vi "IDCheck.vi"(10 "IDIn":u8) -> (2 "IDOut":u8)   [LabVIEW 2013]
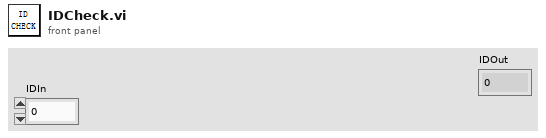
[diagram p1: front panel]
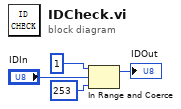
[diagram p0: block diagram]
diagram:
  n1 = In Range and Coerce(upper limit=u8 1, x="IDIn", lower limit=u8 253) -> (coerced(x)=→"IDOut":u8)  [unwired: 1 out]
